vi "poly_time_conversion_ms2s_array.vi"(2 "ms":i32[](array[numeric])) -> (7 "s":dbl[](array[numeric]) format="%#_13g")   [LabVIEW 2015]
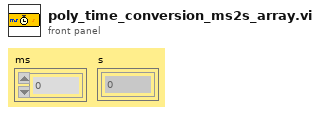
[diagram p1: front panel]
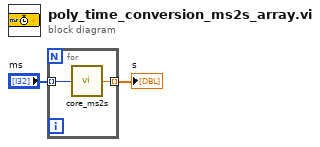
[diagram p0: block diagram]
diagram:
  n1 = for {
    tunnel: "ms" -> [w4] mode=indexing
    tunnel: [w3] -> w1 mode=indexing
    n2 = call "core_ms2s.vi"("ms"=w4) -> ("s"=w3:dbl)  [unwired: 8 in]
  }
  "s" <- w1
